vi "ATS_Spec_List.vi"(11 "Controls[]":refnum<vi>[](array[refnum])) -> (1 "Complete_List":string[](array[string]), 2 "Disabled Items":i32[](array[numeric]), 3 "Selected_Item":string[](array[string]))   [LabVIEW 2015]
doc: "_____AlazarTech, Scope_____\n\nCreate an array list of the Input Control."
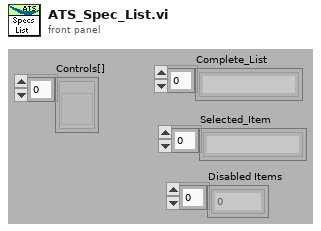
[diagram p1: front panel]
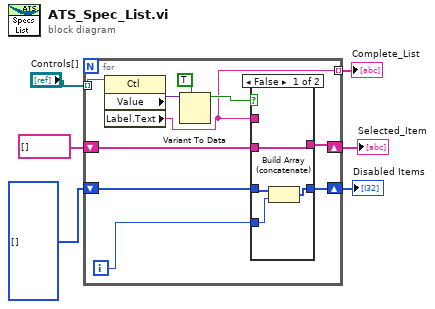
[diagram p0: block diagram]
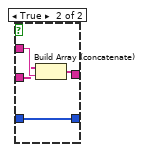
[diagram p2: hidden frame]
diagram:
  n1 = for {
    tunnel: "Controls[]" -> [w16] mode=indexing
    shift-right: [w11] -> w4
    shift-left: string[] [] -> [w13]
    shift-right: [w9] -> w2
    shift-left: i32[] [] ("Disabled Items []") -> [w10]
    tunnel: [w7] -> w1 mode=indexing
    i -> [w8]
    n2 = property class="Ctl"(reference=w16) -> ("Value"=w15:variant, "Label.Text"=w7:string)  [unwired: 1 in, 2 out]
    n3 = Variant To Data(type=TRUE, Variant=w15) -> (data=w12:bool)  [unwired: 1 in, 1 out]
    n4 = case shown="False" w12 {
      tunnel: w13 -> [w20 w23]
      tunnel: [w20 w22] -> w11
      tunnel: w7 -> [_ w24]
      tunnel: w10 -> [w19 w21]
      tunnel: [w17 w21] -> w9
      tunnel: w8 -> [w18 _]
      frame False {
        n5 = Build Array (concatenate)(w19, w18) -> (w17:i32[])
      }
      frame True {
        n6 = Build Array (concatenate)(w23, w24) -> (w22:string[])
      }
    }
  }
  "Selected_Item" <- w4
  "Disabled Items" <- w2
  "Complete_List" <- w1
